vi "Find One by ID.vi"(7 "Entity ID":T1, 8 "error in (no error)":errorcluster, 9 "Entity Definition":refnum<class "Type.lvclass">[](array[class]), 10 "Table Name":string, 11 "Database in":refnum<class "Database Platform.lvclass">) -> (0 "error out":errorcluster, 2 "Result Row":refnum<class "Result Row.lvclass">, 3 "Database out":refnum<class "Database Platform.lvclass">)   [LabVIEW 2022 SP3, in "Conditum.lvlib" / "Database Platform.lvclass"]
uses:
  Database Platform.lvclass
  Database Platform.lvclass/Database Platform.ctl
  Columns/Type/Type.lvclass
  Result Row/Result Row.lvclass
  Entity ID.ctl
  Conditum.lvlib
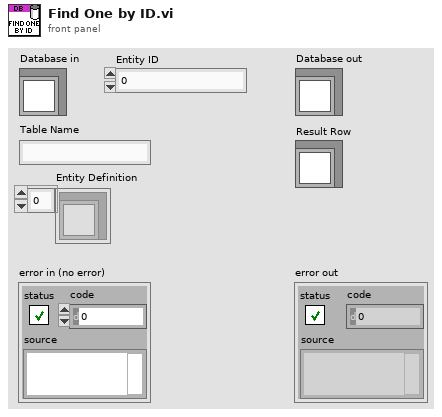
[diagram p1: front panel]
types:
  T1 = typedef "Conditum.lvlib/Entity ID.ctl" = i64
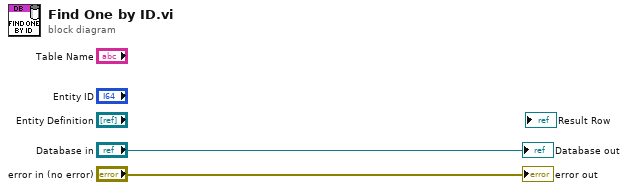
[diagram p0: block diagram]
diagram:
  "error out" <- "error in (no error)"
  "Database out" <- "Database in"
